vi "iniCfg.vi"(8 "error out":errorcluster, 11 "connection ID":refnum<k5>) -> (0 "error out 2":errorcluster caption="error out", 3 "connection ID 2":refnum<k5>)   [LabVIEW 2015]
panel:
  out "문자열":string
  out "문자열 2":string
  out "원소":string
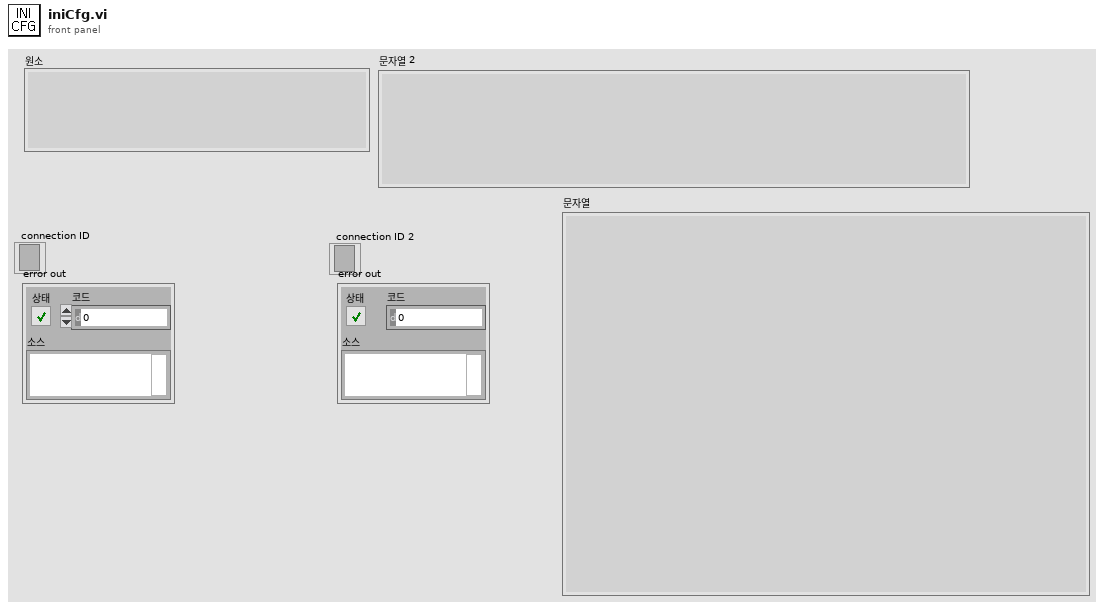
[diagram p1: front panel]
types:
  T1 = enum16{"Standard", "Buffered", "CRLF", "Immediate"}
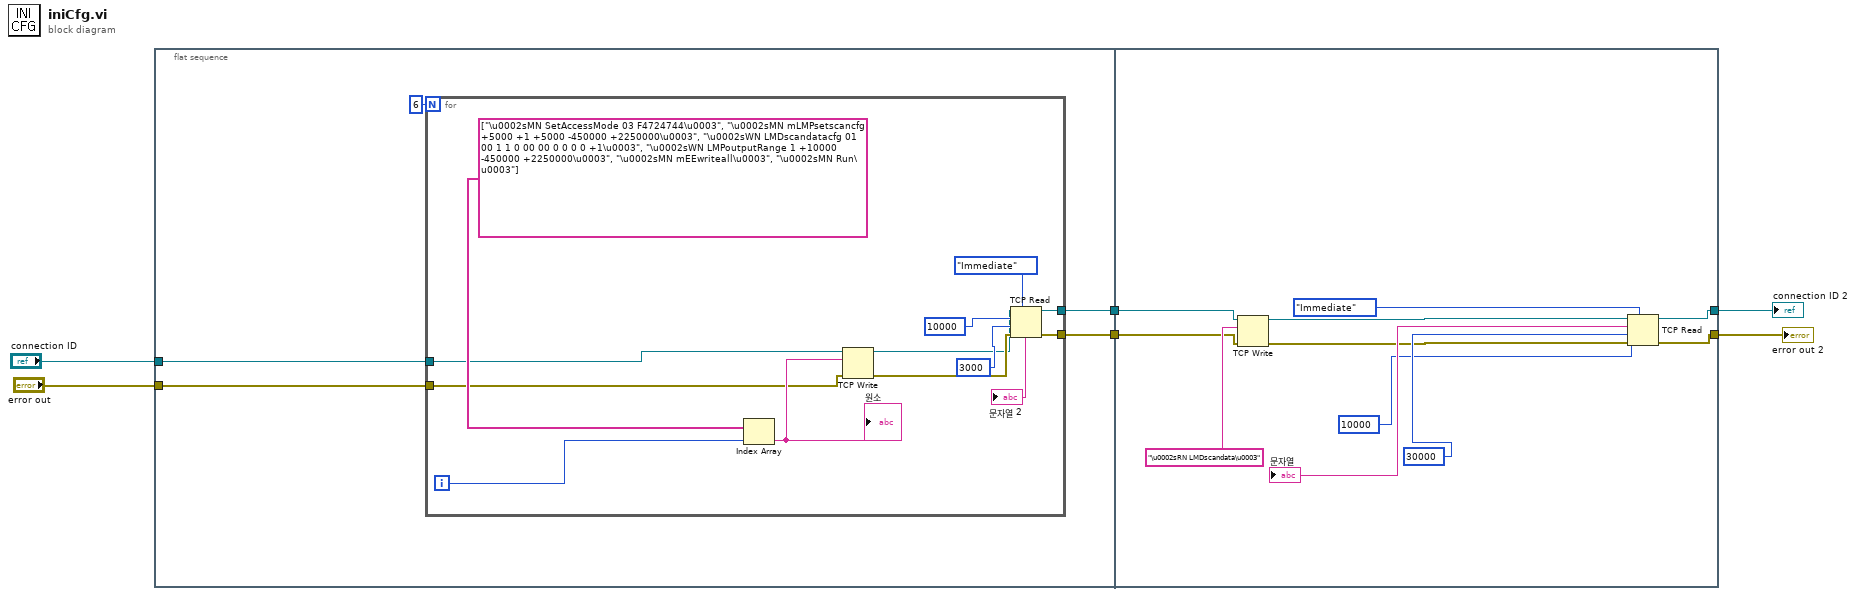
[diagram p0: block diagram]
diagram:
  n1 = flat-sequence {
    tunnel: [w11] -> w4
    tunnel: [w10] -> w3
    tunnel: "error out" -> [w8]
    tunnel: "connection ID" -> [w7]
    tunnel: [w25] -> w5
    tunnel: [w26] -> w6
    tunnel: w4 -> [w28]
    tunnel: w3 -> [w27]
    frame #0 {
      n2 = for {
        N: 6 -> [_]
        tunnel: [w16] -> w11
        tunnel: [w15] -> w10
        tunnel: w8 -> [w13]
        tunnel: w7 -> [w12]
        i -> [w14]
        n3 = Index Array(array=string[] ["\u0002sMN SetAccessMode 03 F4724744\u0003", "\u0002sMN mLMPsetscancfg +5000 +1 +5000 -450000 +2250000\u0003", "\u0002sWN LMDscandatacfg 01 00 1 1 0 00 00 0 0 0 0 +1\u0003", "\u0002sWN LMPoutputRange 1 +10000 -450000 +2250000\u0003", "\u0002sMN mEEwriteall\u0003", "\u0002sMN Run\u0003"], index=w14) -> (element=w19:string)
        "원소" <- w19
        n4 = TCP Write(connection ID=w12, data in=w19, error in (no error)=w13) -> (connection ID out=w17:refnum<k5>, error out=w18:errorcluster)  [unwired: 1 in, 1 out]
        n5 = TCP Read(connection ID=w17, bytes to read=10000 ("읽을 바이트"), error in (no error)=w18, 7:T1."Immediate" ("모드(standard)"), 9:3000 ("타임아웃 ms (25000)")) -> (connection ID out=w16:refnum<k5>, data out=→"문자열 2":string, error out=w15:errorcluster)
      }
    }
    frame #1 {
      n6 = TCP Write(connection ID=w28, data in="\u0002sRN LMDscandata\u0003", error in (no error)=w27) -> (connection ID out=w35:refnum<k5>, error out=w29:errorcluster)  [unwired: 1 in, 1 out]
      n7 = TCP Read(connection ID=w35, bytes to read=10000 ("읽을 바이트"), error in (no error)=w29, 7:T1."Immediate" ("모드(standard)"), 9:30000 ("타임아웃 ms (25000)")) -> (connection ID out=w26:refnum<k5>, data out=→"문자열":string, error out=w25:errorcluster)
    }
  }
  "connection ID 2" <- w6
  "error out 2" <- w5
